vi "Remove Stale Logs.vi"(8 "error in (no error)":errorcluster, 10 "Bad Log?":bool, 11 "Aggregate Logs In":refnum<data-value>) -> (0 "error out":errorcluster, 3 "Aggregate Logs Out":refnum<data-value>)   [LabVIEW 2019, in "Composed Log.lvlib" / "LoggerReference.lvclass"]
uses:
  LoggerReference.lvclass
  Types/MessageCluster.ctl
  Composed Log.lvlib
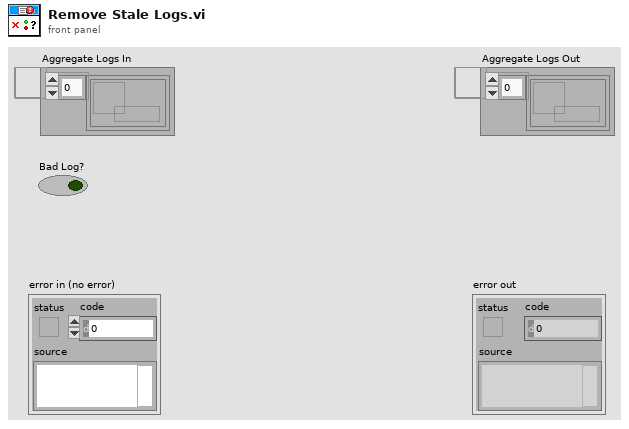
[diagram p1: front panel]
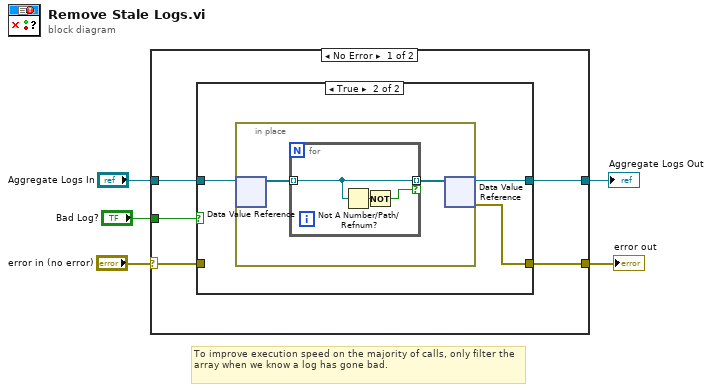
[diagram p0: block diagram]
diagram:
  # "To improve execution speed on the majority of calls, only filter the array when we know a log has gone bad."
  n1 = case shown="No Error" "error in (no error)" {
    selector: "error in (no error)" -> [w7 w22]
    tunnel: "Bad Log?" -> [w10 _]
    tunnel: "Aggregate Logs In" -> [w9 w21]
    tunnel: [w8 w22] -> w2
    tunnel: [w6 w21] -> w1
    frame No Error {
      n2 = case shown="True" w10 {
        tunnel: w9 -> [w11 w15]
        tunnel: [w12 w14] -> w8
        tunnel: w7 -> [w12 _]
        tunnel: [w11 w13] -> w6
        frame False {
        }
        frame True {
          n3 = in-place {
            n4 = in-place-dvr #1(w15) -> (w17:refnum<queue>[])  [unwired: 1 out]
            n5 = for {
              tunnel: w17 -> [w20] mode=indexing
              tunnel: [w20] -> w16 mode=indexing if=w18
              n6 = Not A Number/Path/Refnum?(number/path/refnum=w20) -> (NaN/Path/Refnum?=w19:bool)
              n7 = Not(x=w19) -> (.not. x?=w18:bool)
            }
            n8 = in-place-dvr #1(w16) -> (w13:refnum<data-value>, w14:errorcluster)
          }
        }
      }
    }
    frame Error {
    }
  }
  "error out" <- w2
  "Aggregate Logs Out" <- w1
